vi "Main.vi"() -> ()   [LabVIEW 2020, in "WebServiceImporter.lvlib" / "Main Panel.lvlib" / "Authentication.lvlib"]
uses:
  <vilib>/Platform/WebService/Main Panel/Pages/Authentication/Authentication.lvlib
  <vilib>/Platform/WebService/Main Panel/Pages/Authentication/Events/Events.lvlib
  <vilib>/Platform/WebService/ProxyDll Generator/ProxyDll Generator.lvlib
  <vilib>/Platform/WebService/Main Panel/Main Panel.lvlib
  <vilib>/Platform/WebService/Error Handling/Error Handling.lvlib
  <vilib>/Platform/WebService/Main Panel/Events/Events.lvlib
panel:
  in  "Panel":enum32{"Interface Frame", "Hidden Controls"}(tab)
  in  "Proxy Domain":string caption="Domain"
  in  "Proxy Password":string caption="Password"
  in  "Proxy User Name":string caption="User name*"
  in  "Proxy authentication?":bool
  in  "Port":u32
  in  "Name/Address*":string
  in  "Proxy server?":bool
  in  "Domain":string
  in  "Password":string
  in  "User name*":string
  in  "Web authentication":bool
  # "Input the authentication information"
  # "Authentication"
  # "Proxy Server"
  # "* Marked items are required when the option is enabled."
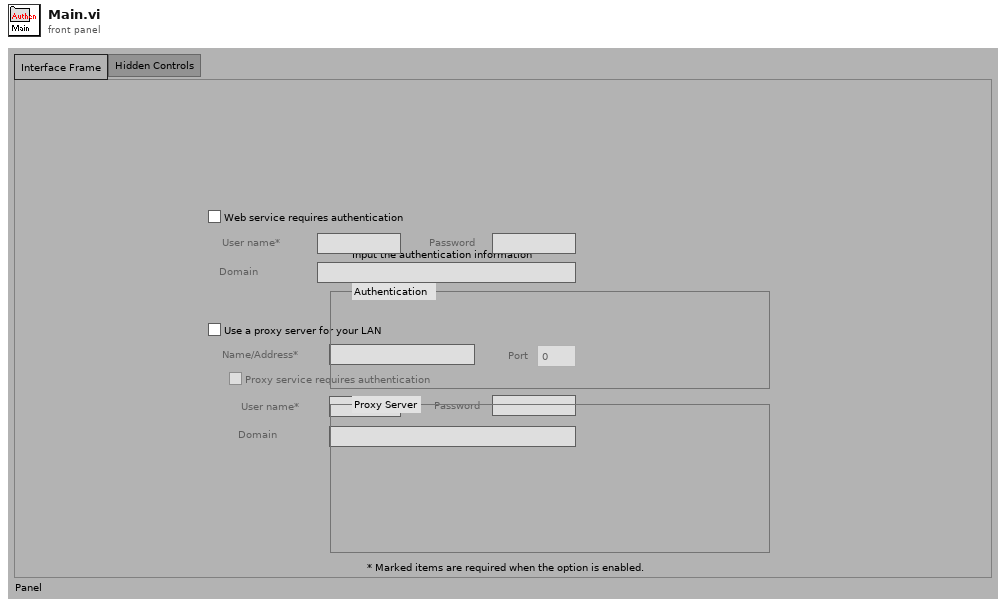
[diagram p1: front panel]
types:
  T1 = cluster{"Use Proxy Server":bool, "Address":string, "Port":u32}
  T2 = cluster{"Need Authentication":bool, "Username":string, "Password":string, "Domain":string}
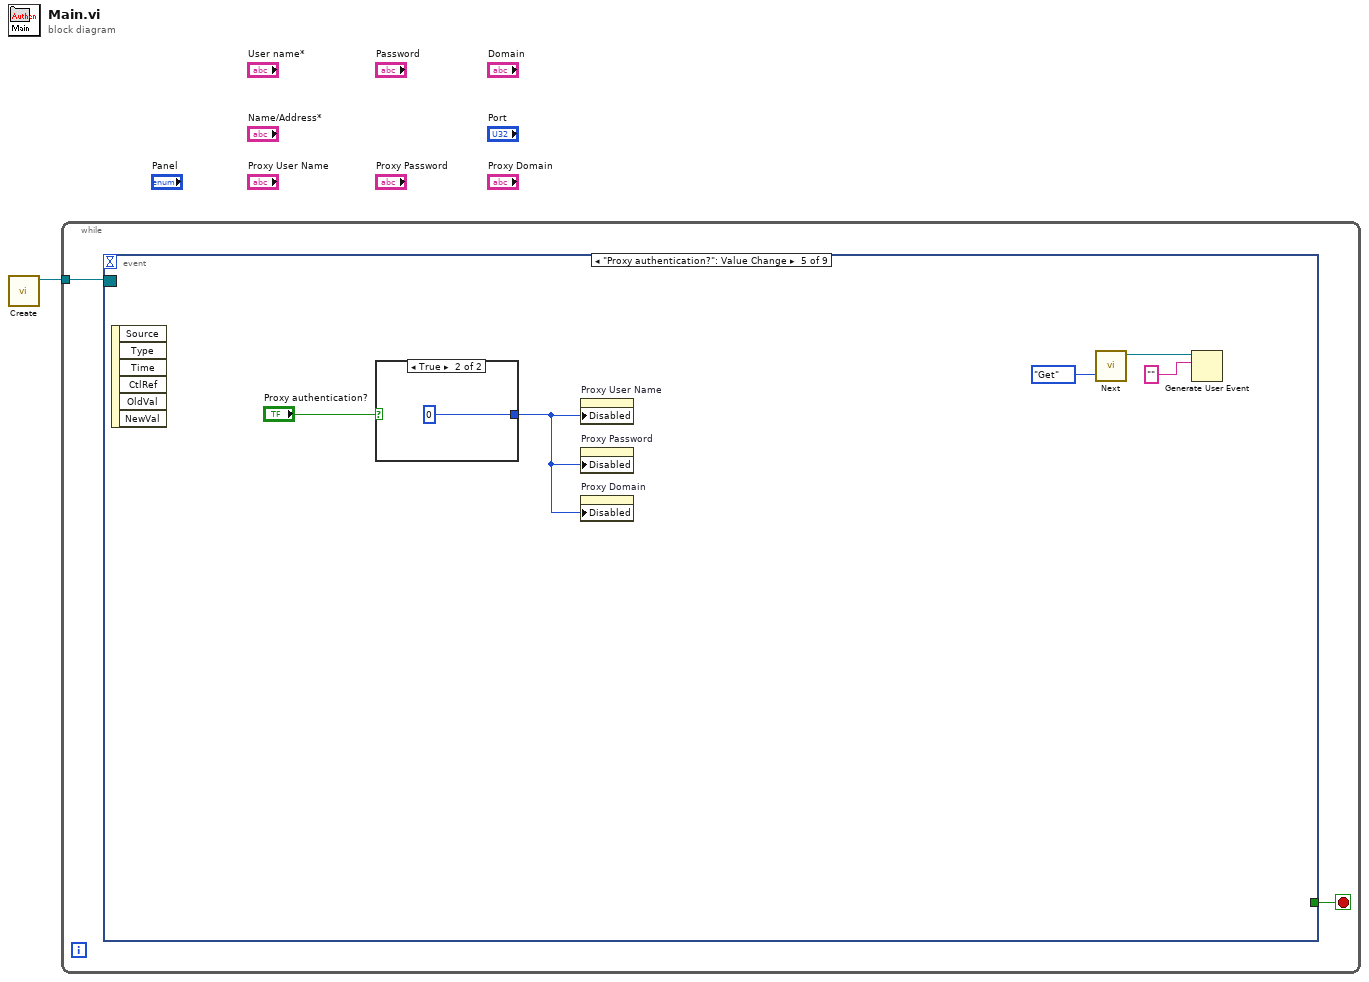
[diagram p0: block diagram]
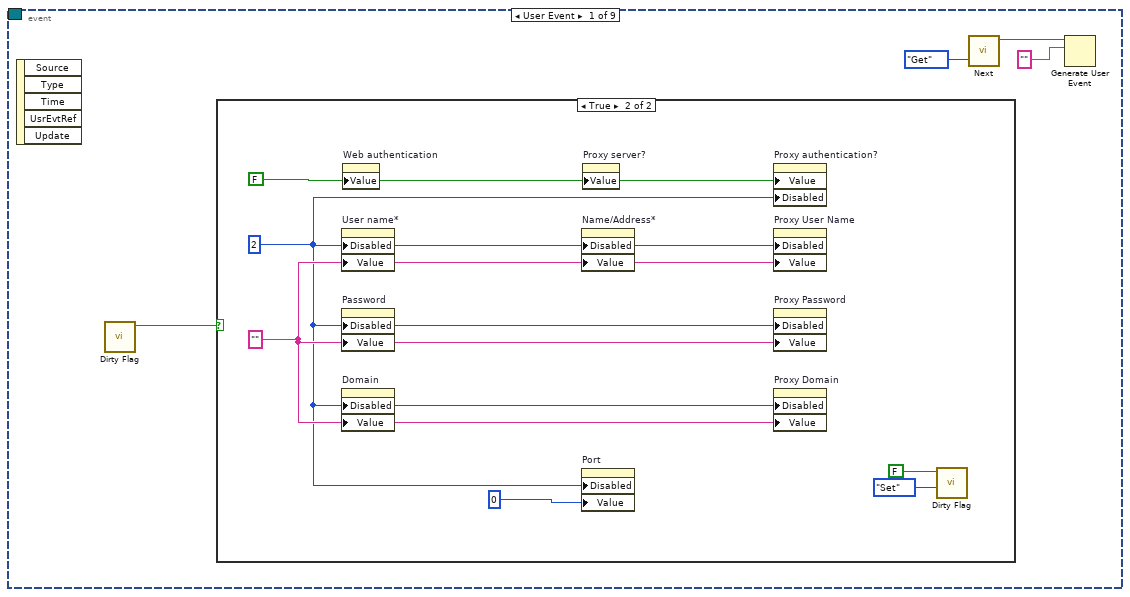
[diagram p2: hidden frame]
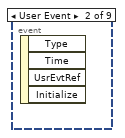
[diagram p4: hidden frame]
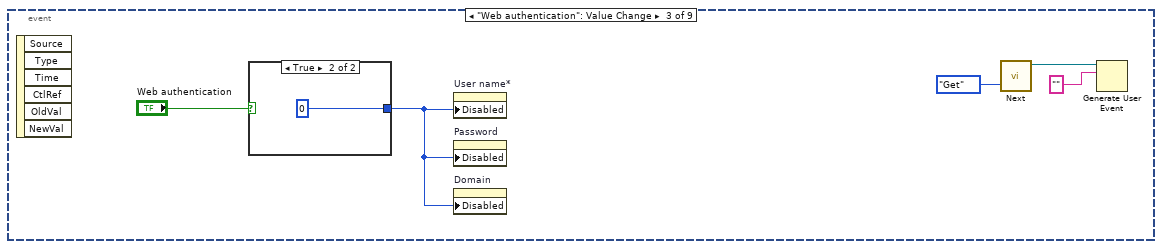
[diagram p5: hidden frame]
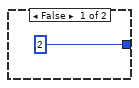
[diagram p6: hidden frame]
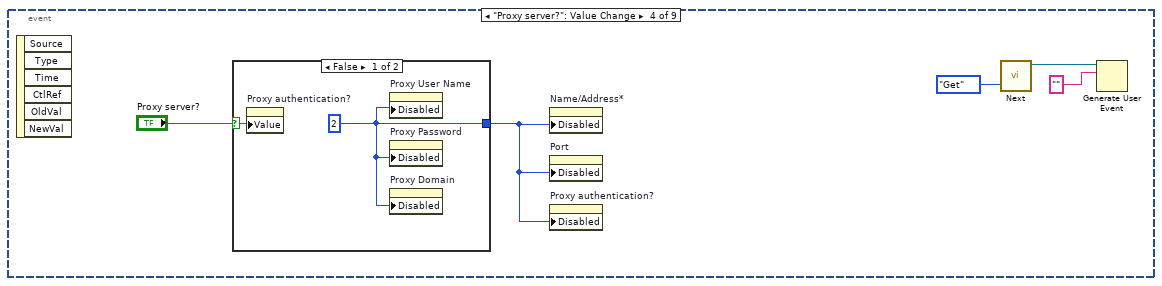
[diagram p7: hidden frame]
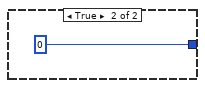
[diagram p8: hidden frame]
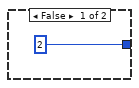
[diagram p9: hidden frame]
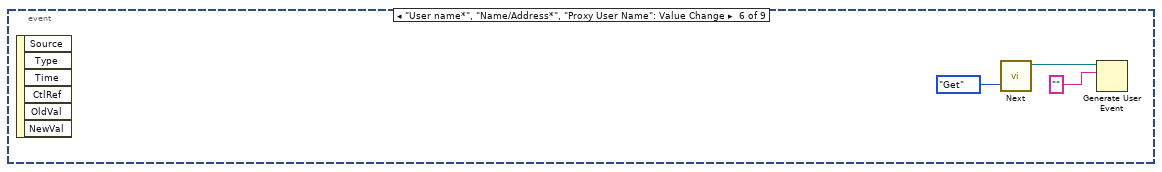
[diagram p10: hidden frame]
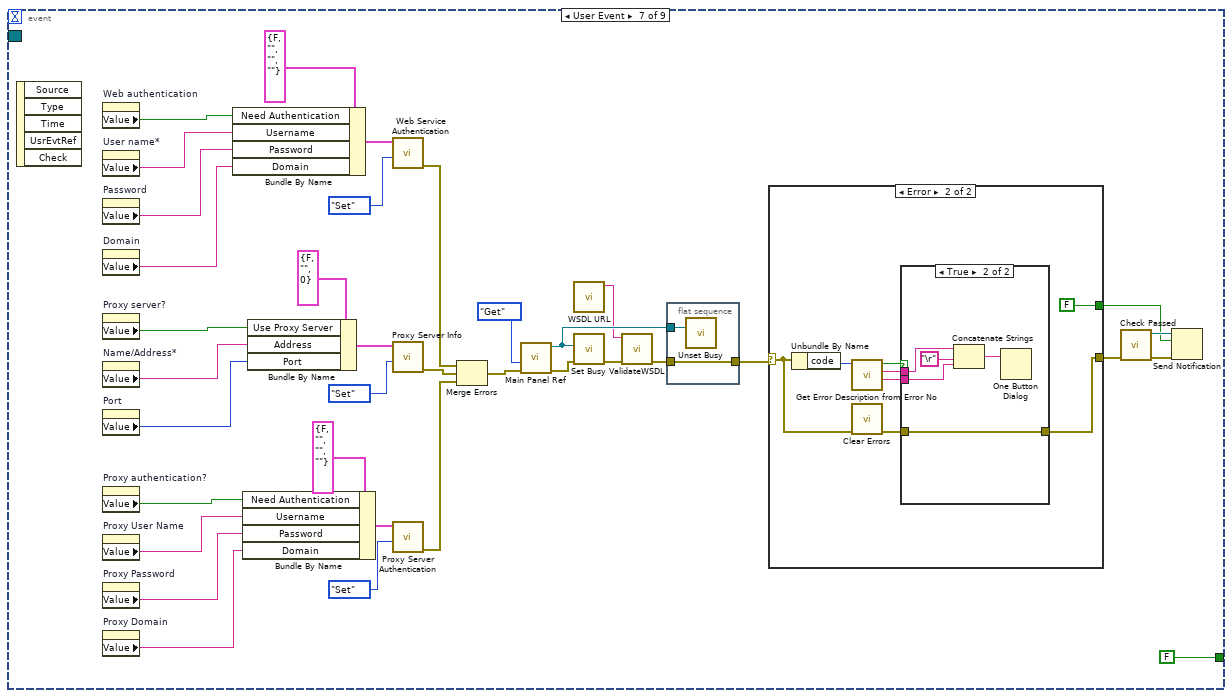
[diagram p11: hidden frame]
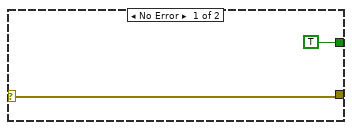
[diagram p12: hidden frame]
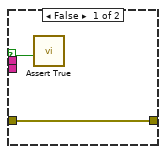
[diagram p13: hidden frame]
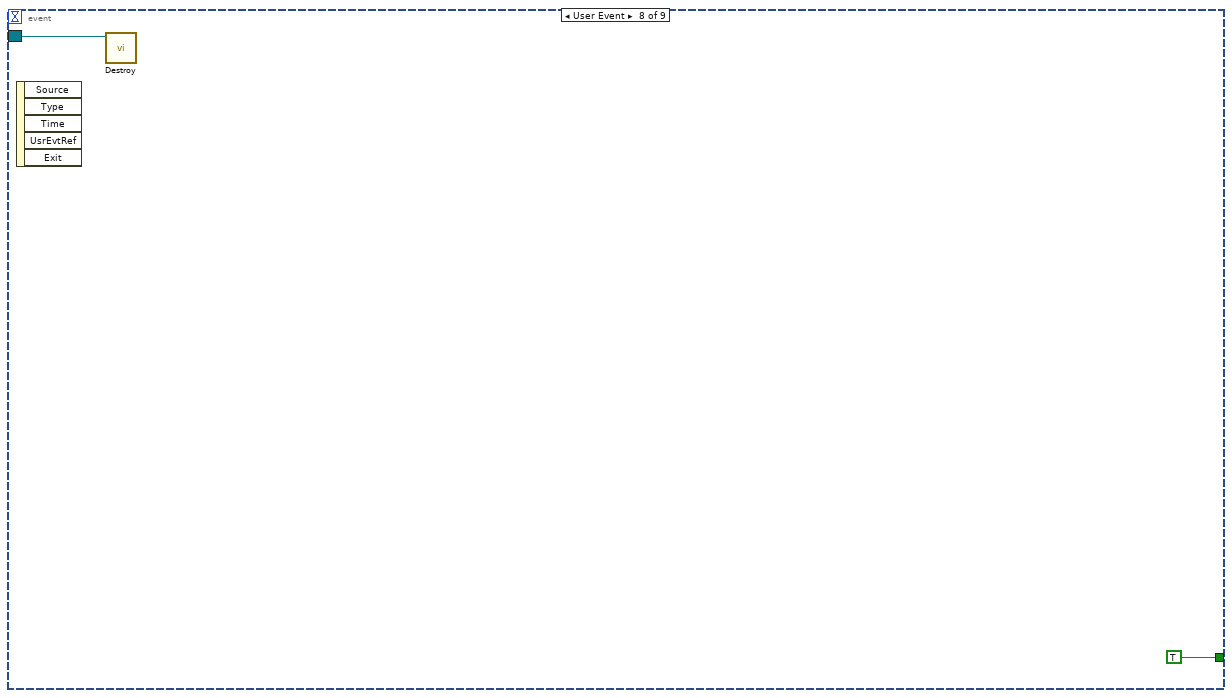
[diagram p14: hidden frame]
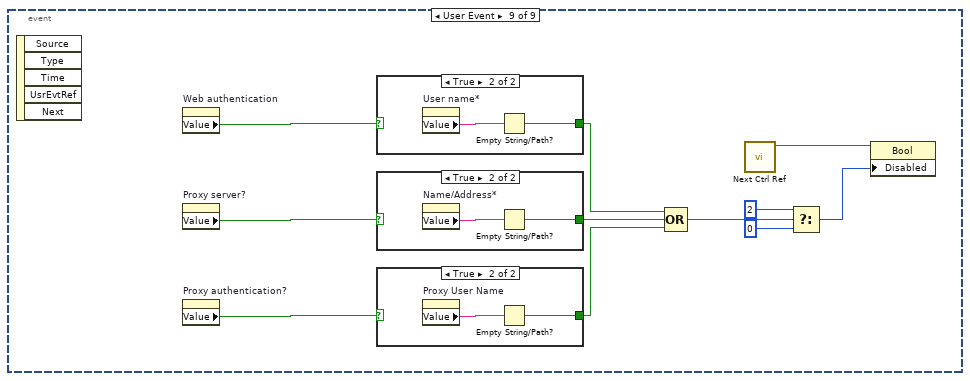
[diagram p15: hidden frame]
diagram:
  n1 = call <vilib>:"Create.vi"() -> ("Event Registration Refnum"=w1:refnum<event-registration>)  [unwired: 1 in, 10 out]
  n2 = while {
    tunnel: w1 -> [w3]
    stop <- w2 stop-if-true
    n3 = event shown="[4] \"Proxy authentication?\": Value Change" {
      selector: w3 -> [_ _ _ _ _ _ _ w94 _]
      dyn-events: _ -> [_ _ _ _ _ _ _ _ _]
      timeout: _ -> [_ _ _ _ _ _ _ _ _]
      tunnel: [_ _ _ _ _ _ FALSE TRUE _] -> w2
      event User Event {
        n4 = event-data() -> ()  [unwired: 6 out]
        n5 = call <vilib>:"Dirty Flag.vi"() -> ("Dirty (out)"=w7:bool)  [unwired: 3 in, 8 out]
        n6 = case shown="True" w7 {
          frame False {
          }
          frame True {
            w11 = ""
            w12 = FALSE ("Web authentication")
            w10 = u8 2
            n7 = property on="User name*" class="Str"("Disabled"=w10, "Value"=w11) -> ()  [unwired: 2 in, 2 out]
            n8 = property on="Password" class="Str"("Disabled"=w10, "Value"=w11) -> ()  [unwired: 2 in, 2 out]
            n9 = property on="Domain" class="Str"("Disabled"=w10, "Value"=w11) -> ()  [unwired: 2 in, 2 out]
            n10 = property on="Web authentication" class="Bool (strict)"("Value"=w12) -> ()  [unwired: 2 in, 2 out]
            n11 = property on="Name/Address*" class="Str"("Disabled"=w10, "Value"=w11) -> ()  [unwired: 2 in, 2 out]
            n12 = property on="Port" class="DigNum (strict)"("Disabled"=w10, "Value"=u32 0 ("Port")) -> ()  [unwired: 2 in, 2 out]
            n13 = property on="Proxy server?" class="Bool (strict)"("Value"=w12) -> ()  [unwired: 2 in, 2 out]
            n14 = property on="Proxy authentication?" class="Bool (strict)"("Value"=w12, "Disabled"=w10) -> ()  [unwired: 2 in, 2 out]
            n15 = property on="Proxy User Name" class="Str"("Disabled"=w10, "Value"=w11) -> ()  [unwired: 2 in, 2 out]
            n16 = property on="Proxy Password" class="Str"("Disabled"=w10, "Value"=w11) -> ()  [unwired: 2 in, 2 out]
            n17 = property on="Proxy Domain" class="Str"("Disabled"=w10, "Value"=w11) -> ()  [unwired: 2 in, 2 out]
            n18 = call <vilib>:"Dirty Flag.vi"("Operation"=enum16{"Get", "Set"}."Set", "Dirty"=FALSE) -> ()  [unwired: 1 in, 9 out]
          }
        }
        n19 = call <vilib>:"Next.vi"("Operation"=enum16{"Get", "Set"}."Get") -> ("user event (out)"=w5:refnum<user-event>)  [unwired: 1 in, 9 out]
        n20 = Generate User Event(user event=w5, event data cluster="" ("event data")) -> ()  [unwired: 2 in, 2 out]
      }
      event User Event {
        n21 = event-data() -> ()  [unwired: 5 out]
      }
      event "Web authentication": Value Change {
        n22 = event-data() -> ()  [unwired: 7 out]
        n23 = case shown="True" "Web authentication" {
          tunnel: [u8 2 ("Disabled") u8 0 ("Disabled")] -> w17
          frame False {
          }
          frame True {
          }
        }
        n24 = property on="User name*" class="Str"("Disabled"=w17) -> ()  [unwired: 2 in, 2 out]
        n25 = property on="Password" class="Str"("Disabled"=w17) -> ()  [unwired: 2 in, 2 out]
        n26 = property on="Domain" class="Str"("Disabled"=w17) -> ()  [unwired: 2 in, 2 out]
        n27 = call <vilib>:"Next.vi"("Operation"=enum16{"Get", "Set"}."Get") -> ("user event (out)"=w15:refnum<user-event>)  [unwired: 1 in, 9 out]
        n28 = Generate User Event(user event=w15, event data cluster="" ("event data")) -> ()  [unwired: 2 in, 2 out]
      }
      event "Proxy server?": Value Change {
        n29 = event-data() -> ()  [unwired: 7 out]
        n30 = case shown="False" "Proxy server?" {
          selector: "Proxy server?" -> [w27 _]
          tunnel: [w26 u8 0 ("Disabled")] -> w24
          frame False {
            w26 = u8 2 ("Disabled")
            n31 = property on="Proxy authentication?" class="Bool (strict)"("Value"=w27) -> ()  [unwired: 2 in, 2 out]
            n32 = property on="Proxy User Name" class="Str"("Disabled"=w26) -> ()  [unwired: 2 in, 2 out]
            n33 = property on="Proxy Password" class="Str"("Disabled"=w26) -> ()  [unwired: 2 in, 2 out]
            n34 = property on="Proxy Domain" class="Str"("Disabled"=w26) -> ()  [unwired: 2 in, 2 out]
          }
          frame True {
          }
        }
        n35 = property on="Name/Address*" class="Str"("Disabled"=w24) -> ()  [unwired: 2 in, 2 out]
        n36 = property on="Port" class="DigNum (strict)"("Disabled"=w24) -> ()  [unwired: 2 in, 2 out]
        n37 = property on="Proxy authentication?" class="Bool (strict)"("Disabled"=w24) -> ()  [unwired: 2 in, 2 out]
        n38 = call <vilib>:"Next.vi"("Operation"=enum16{"Get", "Set"}."Get") -> ("user event (out)"=w22:refnum<user-event>)  [unwired: 1 in, 9 out]
        n39 = Generate User Event(user event=w22, event data cluster="" ("event data")) -> ()  [unwired: 2 in, 2 out]
      }
      event "Proxy authentication?": Value Change {
        n40 = event-data() -> ()  [unwired: 7 out]
        n41 = case shown="True" "Proxy authentication?" {
          tunnel: [u8 2 ("Disabled") u8 0 ("Disabled")] -> w32
          frame False {
          }
          frame True {
          }
        }
        n42 = property on="Proxy User Name" class="Str"("Disabled"=w32) -> ()  [unwired: 2 in, 2 out]
        n43 = property on="Proxy Password" class="Str"("Disabled"=w32) -> ()  [unwired: 2 in, 2 out]
        n44 = property on="Proxy Domain" class="Str"("Disabled"=w32) -> ()  [unwired: 2 in, 2 out]
        n45 = call <vilib>:"Next.vi"("Operation"=enum16{"Get", "Set"}."Get") -> ("user event (out)"=w30:refnum<user-event>)  [unwired: 1 in, 9 out]
        n46 = Generate User Event(user event=w30, event data cluster="" ("event data")) -> ()  [unwired: 2 in, 2 out]
      }
      event "User name*", "Name/Address*", "Proxy User Name": Value Change {
        n47 = event-data() -> ()  [unwired: 7 out]
        n48 = call <vilib>:"Next.vi"("Operation"=enum16{"Get", "Set"}."Get") -> ("user event (out)"=w37:refnum<user-event>)  [unwired: 1 in, 9 out]
        n49 = Generate User Event(user event=w37, event data cluster="" ("event data")) -> ()  [unwired: 2 in, 2 out]
      }
      event User Event {
        n50 = event-data() -> ()  [unwired: 6 out]
        n51 = property on="Web authentication" class="Bool (strict)"() -> ("Value"=w72:bool)  [unwired: 2 in, 2 out]
        n52 = property on="User name*" class="Str"() -> ("Value"=w71:string)  [unwired: 2 in, 2 out]
        n53 = property on="Password" class="Str"() -> ("Value"=w70:string)  [unwired: 2 in, 2 out]
        n54 = property on="Domain" class="Str"() -> ("Value"=w69:string)  [unwired: 2 in, 2 out]
        n55 = property on="Proxy server?" class="Bool (strict)"() -> ("Value"=w58:bool)  [unwired: 2 in, 2 out]
        n56 = property on="Name/Address*" class="Str"() -> ("Value"=w57:string)  [unwired: 2 in, 2 out]
        n57 = property on="Port" class="DigNum (strict)"() -> ("Value"=w56:u32)  [unwired: 2 in, 2 out]
        n58 = property on="Proxy authentication?" class="Bool (strict)"() -> ("Value"=w65:bool)  [unwired: 2 in, 2 out]
        n59 = property on="Proxy User Name" class="Str"() -> ("Value"=w64:string)  [unwired: 2 in, 2 out]
        n60 = property on="Proxy Password" class="Str"() -> ("Value"=w63:string)  [unwired: 2 in, 2 out]
        n61 = property on="Proxy Domain" class="Str"() -> ("Value"=w62:string)  [unwired: 2 in, 2 out]
        n62 = Bundle By Name(cluster=T2 {"Need Authentication"=FALSE, "Username"="", "Password"="", "Domain"=""} ("Web Service Authentication 2"), "Need Authentication"=w72, "Username"=w71, "Password"=w70, "Domain"=w69) -> (w68:T2)
        n63 = Bundle By Name(cluster=T2 {"Need Authentication"=FALSE, "Username"="", "Password"="", "Domain"=""} ("Web Service Authentication 2"), "Need Authentication"=w65, "Username"=w64, "Password"=w63, "Domain"=w62) -> (w61:T2)
        n64 = Bundle By Name(cluster=T1 {"Use Proxy Server"=FALSE, "Address"="", "Port"=0} ("Proxy Server Info"), "Use Proxy Server"=w58, "Address"=w57, "Port"=w56) -> (w55:T1)
        n65 = call <vilib>:"Web Service Authentication.vi"("Get/Set"=enum16{"Get", "Set"}."Set", "Web Service Authentication"=w68) -> ("error out"=w42:errorcluster)  [unwired: 1 in, 8 out]
        n66 = call <vilib>:"Proxy Server Info.vi"("Get/Set"=enum16{"Get", "Set"}."Set", "Proxy Server Info"=w55) -> ("error out"=w41:errorcluster)  [unwired: 1 in, 8 out]
        n67 = call <vilib>:"Proxy Server Authentication.vi"("Get/Set"=enum16{"Get", "Set"}."Set", "Web Service Authentication"=w61) -> ("error out"=w40:errorcluster)  [unwired: 1 in, 8 out]
        n68 = Merge Errors(w42, w41, w40) -> (w43:errorcluster)
        n69 = call <vilib>:"Main Panel Ref.vi"("error in (no error)"=w43, "Operation"=enum16{"Get", "Set"}."Get") -> ("error out"=w44:errorcluster, "VI Refnum (out)"=w52:refnum<vi>)  [unwired: 1 in, 7 out]
        n70 = call <vilib>:"WSDL URL.vi"() -> ("WSDL URL (out)"=w39:string)  [unwired: 3 in, 8 out]
        n71 = call <vilib>:"Set Busy.vi"("error in (no error)"=w44, "VI reference (current VI)"=w52) -> ("error out"=w53:errorcluster)  [unwired: 2 in, 7 out]
        n72 = call <vilib>:"ValidateWSDL.vi"("error in (no error)"=w53, "WSDL URL"=w39) -> ("error out"=w51:errorcluster)  [unwired: 9 out]
        n73 = flat-sequence {
          tunnel: w52 -> [w93]
          tunnel: w51 -> [w92]
          tunnel: [w92] -> w50
          frame #0 {
            n74 = call <vilib>:"Unset Busy.vi"("VI reference (current VI)"=w93) -> ()  [unwired: 1 in, 10 out]
          }
        }
        n75 = case shown="Error" w50 {
          selector: w50 -> [w75 w80]
          tunnel: [w75 w78] -> w47
          tunnel: [TRUE ("notification") FALSE ("notification")] -> w46
          frame No Error {
          }
          frame Error {
            n76 = Unbundle By Name(w80) -> ("code"=w84:i32)
            n77 = call <vilib>:"Get Error Description from Error No.vi"("Error Number"=w84) -> ("Error Description"=w81:string, "Error Title"=w82:string, "Found?"=w83:bool)  [unwired: 8 out]
            n78 = call <vilib>:"Clear Errors.vi"("error in (no error)"=w80) -> ("error out"=w79:errorcluster)  [unwired: 1 in, 5 out]
            n79 = case shown="True" w83 {
              selector: w83 -> [w86 _]
              tunnel: w82 -> [_ w91]
              tunnel: w81 -> [_ w89]
              tunnel: w79 -> [w85 w88]
              tunnel: [w85 w88] -> w78
              frame False {
                n80 = call <vilib>:"Assert True.vi"("Boolean ( True)"=w86) -> ()  [unwired: 11 out]
              }
              frame True {
                n81 = Concatenate Strings(w91, "\r", w89) -> (w87:string)
                n82 = One Button Dialog(message=w87) -> ()  [unwired: 2 out]
              }
            }
          }
        }
        n83 = call <vilib>:"Check Passed.vi"("error in (no error)"=w47) -> ("error out"=w49:errorcluster, "notifier  (out)"=w48:refnum<notifier>)  [unwired: 2 in, 7 out]
        n84 = Send Notification(notification=w46, notifier=w48, error in (no error)=w49) -> ()  [unwired: 2 out]
      }
      event User Event {
        n85 = event-data() -> ()  [unwired: 6 out]
        n86 = call <vilib>:"Destroy.vi"("Event Registration Refnum"=w94) -> ()  [unwired: 1 in, 10 out]
      }
      event User Event {
        n87 = event-data() -> ()  [unwired: 6 out]
        n88 = property on="Web authentication" class="Bool (strict)"() -> ("Value"=w101:bool)  [unwired: 2 in, 2 out]
        n89 = property on="Proxy server?" class="Bool (strict)"() -> ("Value"=w103:bool)  [unwired: 2 in, 2 out]
        n90 = property on="Proxy authentication?" class="Bool (strict)"() -> ("Value"=w102:bool)  [unwired: 2 in, 2 out]
        n91 = case shown="True" w101 {
          selector: w101 -> [w113 _]
          tunnel: [w113 w114] -> w104
          frame False {
          }
          frame True {
            n92 = property on="User name*" class="Str"() -> ("Value"=w115:string)  [unwired: 2 in, 2 out]
            n93 = Empty String/Path?(string/path=w115) -> (empty?=w114:bool)
          }
        }
        n94 = case shown="True" w103 {
          selector: w103 -> [w110 _]
          tunnel: [w110 w111] -> w105
          frame False {
          }
          frame True {
            n95 = property on="Name/Address*" class="Str"() -> ("Value"=w112:string)  [unwired: 2 in, 2 out]
            n96 = Empty String/Path?(string/path=w112) -> (empty?=w111:bool)
          }
        }
        n97 = case shown="True" w102 {
          selector: w102 -> [w107 _]
          tunnel: [w107 w108] -> w106
          frame False {
          }
          frame True {
            n98 = property on="Proxy User Name" class="Str"() -> ("Value"=w109:string)  [unwired: 2 in, 2 out]
            n99 = Empty String/Path?(string/path=w109) -> (empty?=w108:bool)
          }
        }
        n100 = Compound Arithmetic op=OR(w104, w105, w106) -> (w97:bool)
        n101 = call <vilib>:"Next Ctrl Ref.vi"() -> ("Ctl Refnum (out)"=w96:refnum<vi>)  [unwired: 3 in, 8 out]
        n102 = Select(t=u8 2 ("Disabled"), s=w97, f=u8 0 ("Disabled")) -> (s? t:f=w100:u8)
        n103 = property class="Bool"(reference=w96, "Disabled"=w100) -> ()  [unwired: 1 in, 2 out]
      }
    }
  }
